vi "Syringe_SendCmd.vi"(8 "error in (no error)":errorcluster, 10 "command":string, 11 "VISA resource name":refnum<visa-resource-name>) -> (0 "error out":errorcluster, 2 "Message":string, 3 "VISA resource out":refnum<visa-resource-name>)   [LabVIEW 2015]
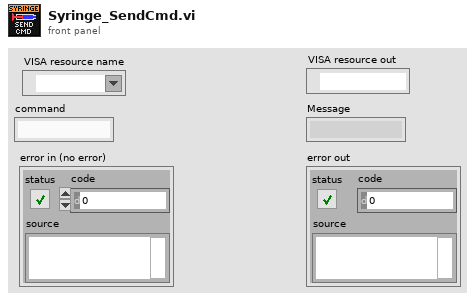
[diagram p1: front panel]
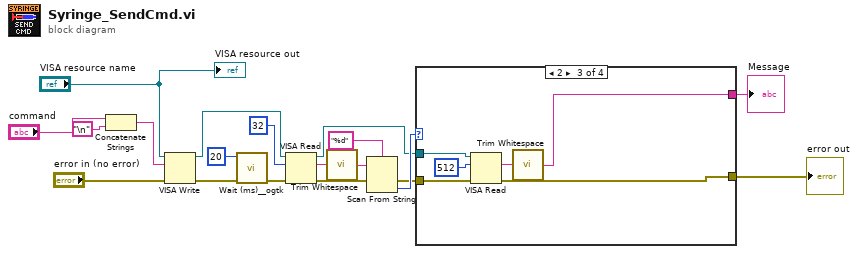
[diagram p0: block diagram]
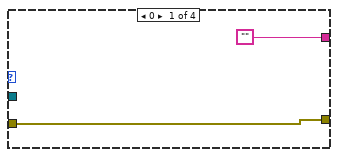
[diagram p2: hidden frame]
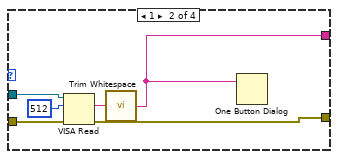
[diagram p3: hidden frame]
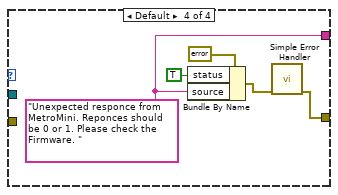
[diagram p4: hidden frame]
diagram:
  n1 = Concatenate Strings("command", "\n") -> (w13:string)
  n2 = VISA Write(VISA resource name="VISA resource name", write buffer=w13, error in (no error)="error in (no error)") -> (VISA resource name out=w14:refnum<visa-resource-name>, error out=w17:errorcluster)  [unwired: 1 out]
  n3 = call <userlib>:"Wait (ms)__ogtk.vi"("error in (no error)"=w17, "milliseconds to wait"=u32 20) -> ("error out"=w15:errorcluster)  [unwired: 8 in, 1 out]
  n4 = VISA Read(VISA resource name=w14, byte count=u32 32, error in (no error)=w15) -> (VISA resource name out=w4:refnum<visa-resource-name>, read buffer=w3:string, error out=w7:errorcluster)  [unwired: 1 out]
  n5 = call <vilib>:"Trim Whitespace.vi"("string"=w3) -> ("trimmed string"=w2:string)  [unwired: 1 in]
  n6 = Scan From String(format string="%d", input string=w2, error in=w7) -> (error out=w6:errorcluster, output 1=w8:i32)  [unwired: 2 in, 2 out]
  n7 = case shown="2" w8 {
    tunnel: w6 -> [w21 w25 w31 _]
    tunnel: [w21 w23 w29 w34] -> w1
    tunnel: ["" w22 w28 w36] -> w5
    tunnel: w4 -> [_ w26 w32 _]
    frame 0 {
    }
    frame 1 {
      n8 = VISA Read(VISA resource name=w26, byte count=u32 512, error in (no error)=w25) -> (read buffer=w24:string, error out=w23:errorcluster)  [unwired: 2 out]
      n9 = call <vilib>:"Trim Whitespace.vi"("string"=w24) -> ("trimmed string"=w22:string)  [unwired: 1 in]
      n10 = One Button Dialog(message=w22) -> ()  [unwired: 1 in, 1 out]
    }
    frame 2 {
      n11 = VISA Read(VISA resource name=w32, byte count=u32 512, error in (no error)=w31) -> (read buffer=w30:string, error out=w29:errorcluster)  [unwired: 2 out]
      n12 = call <vilib>:"Trim Whitespace.vi"("string"=w30) -> ("trimmed string"=w28:string)  [unwired: 1 in]
    }
    frame Default {
      w36 = "Unexpected responce from MetroMini. Reponces should be 0 or 1. Please check the Firmware. " ("source")
      n13 = Bundle By Name(cluster=errorcluster {"status"=FALSE, "code"=0, "source"=""} ("error out 2"), "status"=TRUE, "source"=w36) -> (w35:errorcluster)
      n14 = call <vilib>:"Simple Error Handler.vi"("error in (no error)"=w35) -> ("error out"=w34:errorcluster)  [unwired: 4 in, 4 out]
    }
  }
  "error out" <- w1
  "Message" <- w5
  "VISA resource out" <- "VISA resource name"
